vi "ThrowACard.vi"(10 "SelectedIndex":u16, 11 "Player":T1) -> (3 "NewPlayer":T1)   [LabVIEW 2025]
uses:
  Controls/Player.ctl
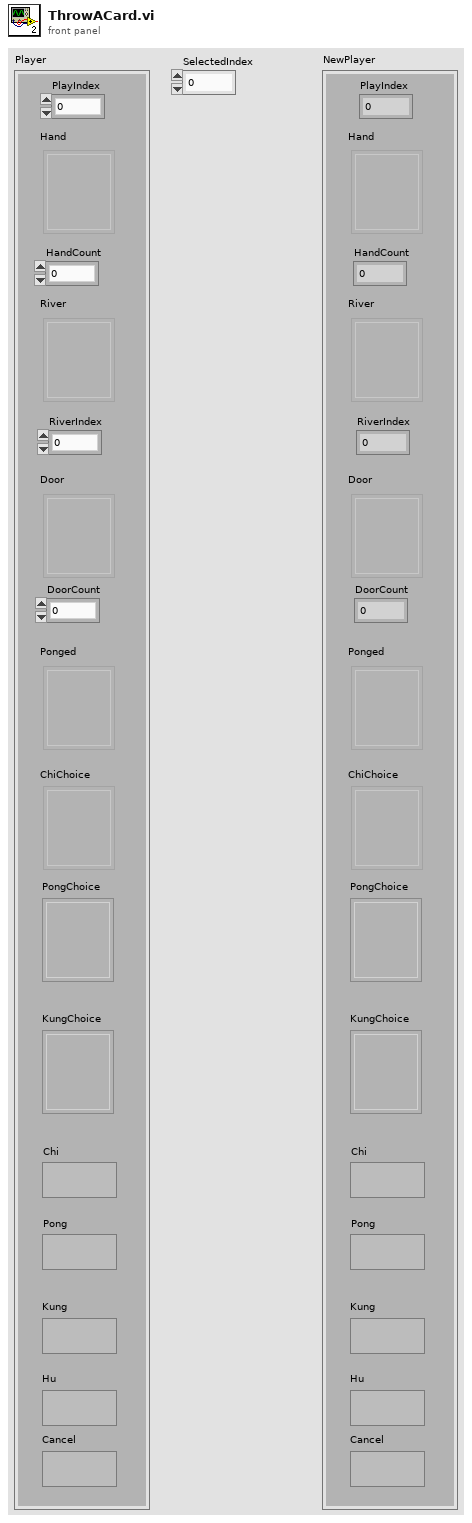
[diagram p1: front panel]
types:
  T1 = typedef "Player.ctl" = cluster{"PlayIndex":u16, "Hand":u16[], "HandCount":u16, "RiverIndex":u16, "Door":u16[], "DoorCount":u16, "Ponged":u16[], "ChiChoice":u16[][], "River":u16[][], "Chi":bool, "Pong":bool, "Kung":bool, "Hu":bool, "Cancel":bool, "PongChoice":u16, "KungChoice":u16}
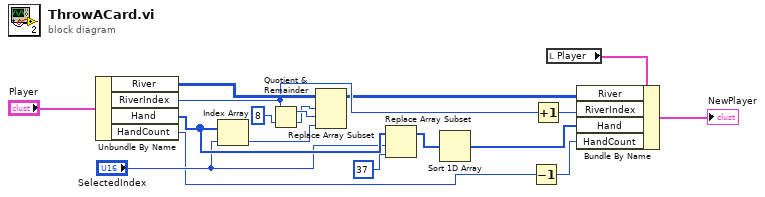
[diagram p0: block diagram]
diagram:
  n1 = Unbundle By Name("Player") -> ("River"=w17:u16[][], "RiverIndex"=w2:u16, "Hand"=w12:u16[], "HandCount"=w4:u16)
  n2 = Index Array(array=w12, index="SelectedIndex") -> (element=w13:u16)
  n3 = Quotient & Remainder(x=w2, y=8) -> (x-y*floor(x/y)=w15:i32, floor(x/y)=w14:i32)
  n4 = Replace Array Subset(array=w17, new element=w13, index (row)=w14, index (col)=w15) -> (w1:u16[][])
  n5 = Replace Array Subset(array=w12, new element=37, index="SelectedIndex") -> (w9:u16[])
  n6 = Sort 1D Array(array=w9) -> (sorted array=w6:u16[])
  n7 = Decrement(x=w4) -> (x-1=w5:u16)
  n8 = Increment(x=w2) -> (x+1=w3:u16)
  n9 = local read "Player"() -> (w7:T1)
  n10 = Bundle By Name(cluster=w7, "River"=w1, "RiverIndex"=w3, "Hand"=w6, "HandCount"=w5) -> (→"NewPlayer":T1)
